vi "CheckTimeoutNotifier.vi"(8 "error in (no error)":errorcluster, 11 "Lockin Error Timeout":refnum<notifier>) -> (0 "error out":errorcluster, 3 "Timeout?":bool)   [LabVIEW 2019, in "AFM_Litho_Plugin.IV.lvclass"]
uses:
  AFM_Litho_Plugin.IV.lvclass
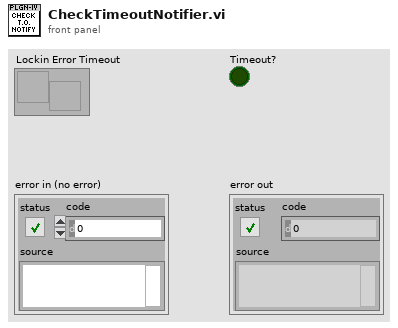
[diagram p1: front panel]
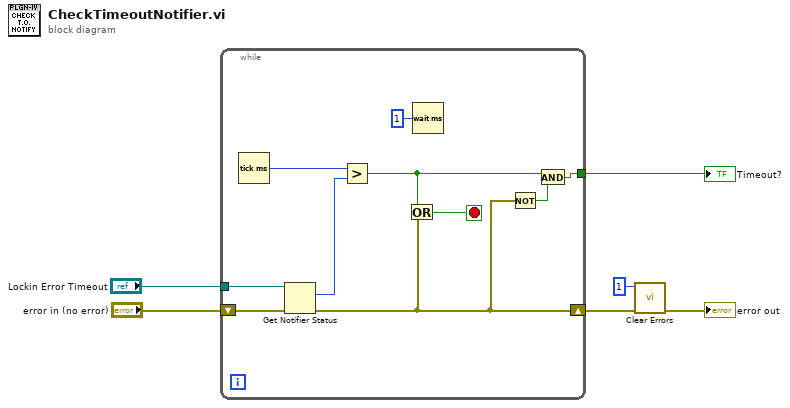
[diagram p0: block diagram]
diagram:
  n1 = while {
    shift-right: [w10] -> w2
    shift-left: "error in (no error)" -> [w16]
    tunnel: "Lockin Error Timeout" -> [w15]
    tunnel: [w7] -> w4
    stop <- w12 stop-if-true
    n2 = Tick Count (ms)() -> (millisecond timer value=w14:u32)
    n3 = Get Notifier Status(notifier=w15, error in (no error)=w16) -> (current notification=w13:u32, error out=w10:errorcluster)  [unwired: 3 out]
    n4 = Greater?(x=w14, y=w13) -> (0:w8:bool)
    n5 = Or(x=w8, y=w10) -> (x .or. y?=w12:bool)
    n6 = Wait (ms)(milliseconds to wait=u32 1) -> ()  [unwired: 1 out]
    n7 = Not(x=w10) -> (.not. x?=w9:bool)
    n8 = And(x=w8, y=w9) -> (x .and. y?=w7:bool)
  }
  "Timeout?" <- w4
  n9 = call <vilib>:"Clear Errors.vi"("error in (no error)"=w2, "specific error code to clear (0: all)"=1) -> ("error out"=→"error out":errorcluster)  [unwired: 4 in, 1 out]
